vi "Pop_up.vi"(0 "Boolean":bool) -> ()   [LabVIEW 2020]
doc: "This Vi is used as a popup vi which is started with an invoke node from the main vi"
panel:
  # "Click this button to stop the execution of the VI"
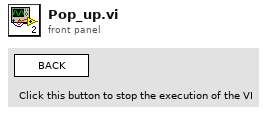
[diagram p1: front panel]
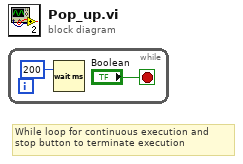
[diagram p0: block diagram]
diagram:
  # "While loop for continuous execution and\nstop button to terminate execution"
  n1 = while {
    stop <- "Boolean" stop-if-true
    n2 = Wait (ms)(milliseconds to wait=u32 200) -> ()  [unwired: 1 out]
  }
